vi "check_generate_new_custom_array.vi"(0 "Cluster":T1, 1 "output values cluster":T2) -> (2 "output cluster":T1, 3 "Need new custom array?":bool, 4 "Output values cluster":T3)   [LabVIEW 2010]
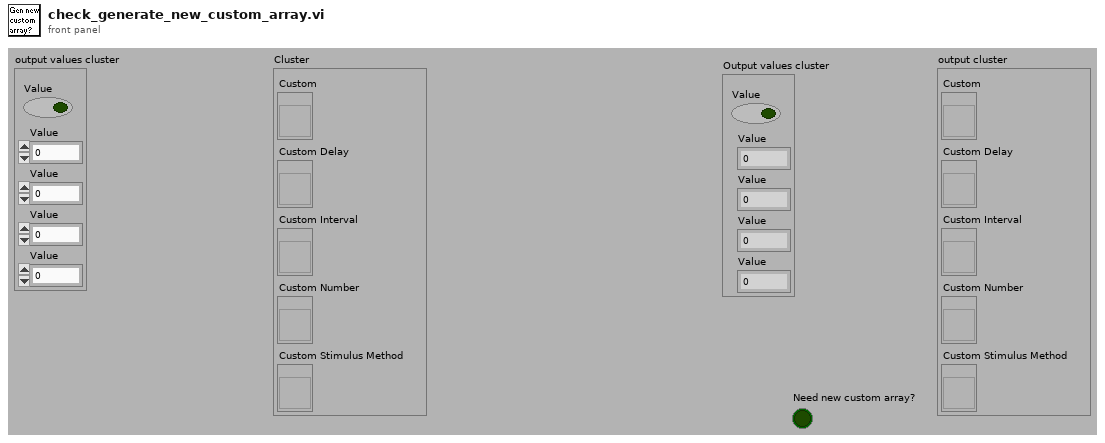
[diagram p1: front panel]
types:
  T1 = cluster{"Custom":refnum<vi>, "Custom Delay":refnum<vi>, "Custom Interval":refnum<vi>, "Custom Number":refnum<vi>, "Custom Stimulus Method":refnum<vi>}
  T2 = cluster{"Value":bool, "Value":dbl, "Value":dbl, "Value":i32, "Value":u16}
  T3 = cluster{"Value":bool, "Value":dbl, "Value":dbl, "Value":dbl, "Value":u16}
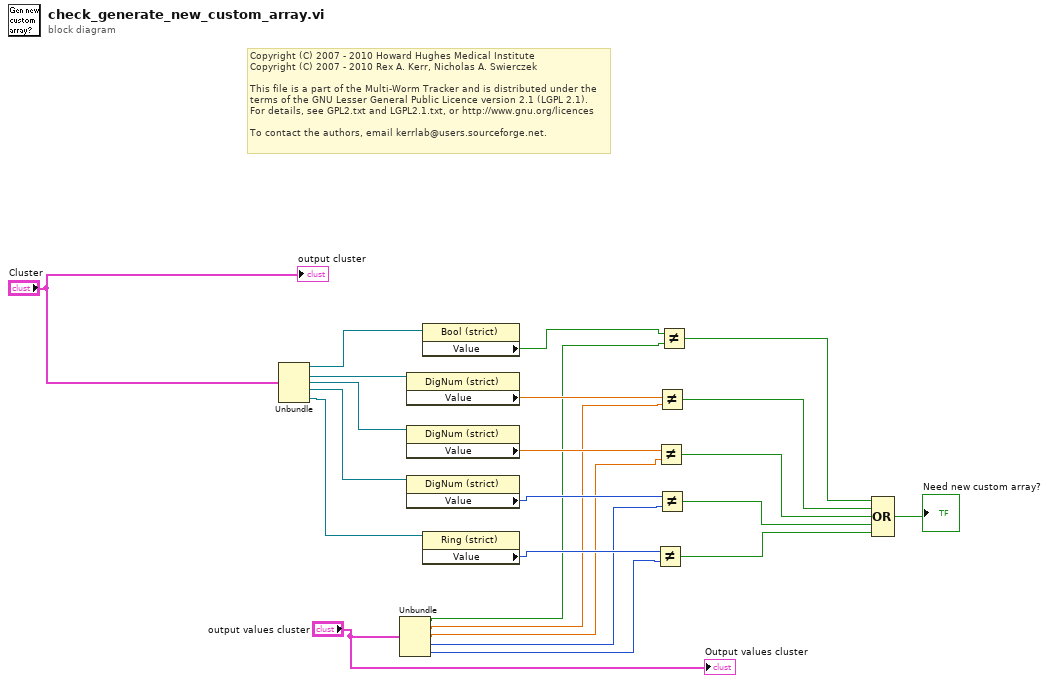
[diagram p0: block diagram]
diagram:
  # "Copyright (C) 2007 - 2010 Howard Hughes Medical Institute\nCopyright (C) 2007 - 2010 Rex A. Kerr, Nicholas A. Swierczek\n \nThis file is a part of the Multi-Worm Tracker and is distributed under the\nterms of the GNU Lesser General Public Licence version 2.1 (LGPL 2.1).\nFor details, see GPL2.txt and LGPL2.1.txt, or http://www.gnu.org/licences\n \nTo contact the authors, email kerrlab@users.sourceforge.net."
  n1 = Unbundle("Cluster") -> ("Custom"=w23:refnum<vi>, "Custom Delay"=w22:refnum<vi>, "Custom Interval"=w21:refnum<vi>, "Custom Number"=w20:refnum<vi>, "Custom Stimulus Method"=w19:refnum<vi>)
  n2 = Unbundle("output values cluster") -> ("Value"=w13:bool, "Value"=w12:dbl, "Value"=w11:dbl, "Value"=w10:i32, "Value"=w9:u16)
  n3 = property class="DigNum (strict)"(reference=w22) -> ("Value"=w17:dbl)  [unwired: 1 in, 2 out]
  n4 = property class="DigNum (strict)"(reference=w21) -> ("Value"=w16:dbl)  [unwired: 1 in, 2 out]
  n5 = property class="DigNum (strict)"(reference=w20) -> ("Value"=w15:i32)  [unwired: 1 in, 2 out]
  n6 = property class="Bool (strict)"(reference=w23) -> ("Value"=w18:bool)  [unwired: 1 in, 2 out]
  n7 = property class="Ring (strict)"(reference=w19) -> ("Value"=w14:u16)  [unwired: 1 in, 2 out]
  n8 = Not Equal?(x=w14, y=w9) -> (x != y?=w4:bool)
  n9 = Not Equal?(x=w16, y=w11) -> (x != y?=w6:bool)
  n10 = Not Equal?(x=w17, y=w12) -> (x != y?=w7:bool)
  n11 = Not Equal?(x=w15, y=w10) -> (x != y?=w5:bool)
  n12 = Not Equal?(x=w18, y=w13) -> (x != y?=w8:bool)
  n13 = Compound Arithmetic op=OR(w8, w7, w6, w5, w4) -> (→"Need new custom array?":bool)
  "Output values cluster" <- "output values cluster"
  "output cluster" <- "Cluster"
